vi "Show User Interface.vi"(8 "error in (no error)":errorcluster, 9 "Process VI Refnums":refnum<vi>[](array[refnum]), 10 "Show UI":bool, 11 "SMO.UI":refnum<class "SMO.UI.lvclass">) -> (0 "error out":errorcluster, 3 "SMO.UI out":refnum<class "SMO.UI.lvclass">)   [LabVIEW 2019, in "SMO.UI.lvclass"]
doc: "JKI State Machine Objects (SMO) 1.3.0.56\nJKI - JKI\nCopyright (c) 2017, JKI"
uses:
  SMO.UI.lvclass
  C:/Users/Patrick/Documents/GitHub/Test (LV2019)/lv-venv/lv.lib/vi.lib/JKI/JKI SMO/SMO/SMO.lvclass
  SMO/SMO.lvclass
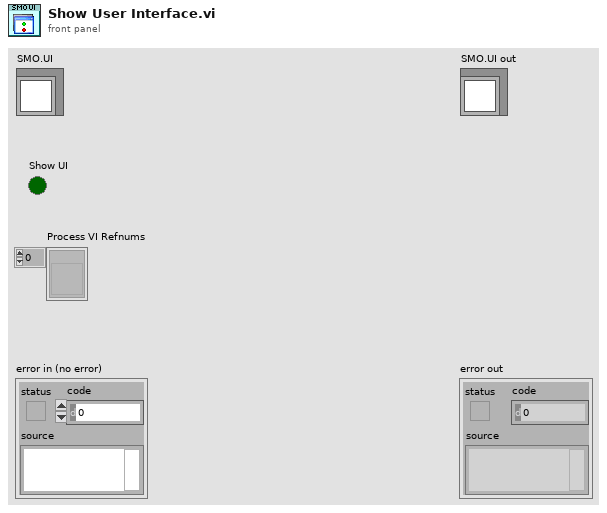
[diagram p1: front panel]
types:
  T1 = enum32{"Invalid", "Standard", "Closed", "Hidden", "Minimized", "Maximized"}
  T2 = typedef "SMO.lvclass/RegisteredProcessData--Cluster.ctl" = cluster{"Name":string, "Static VI Ref":refnum<vi>, "Running":bool, "NotifierRef":u32}
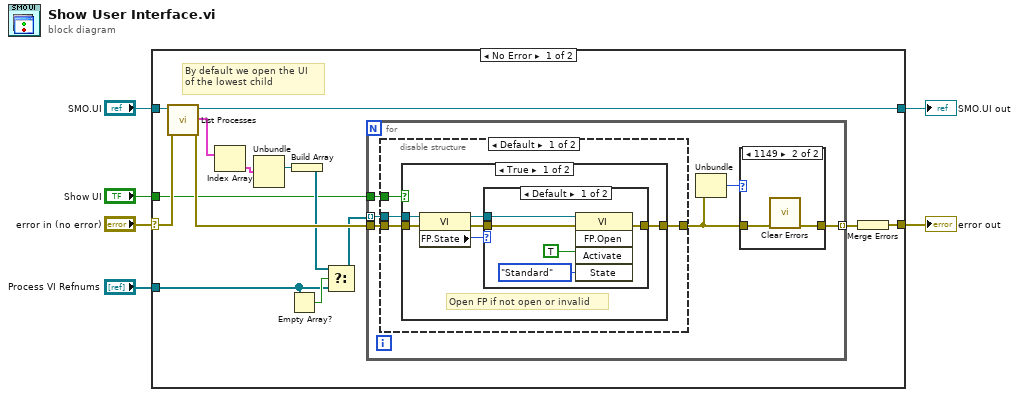
[diagram p0: block diagram]
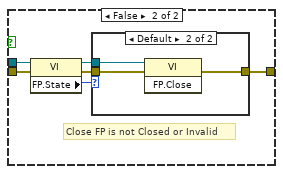
[diagram p4: hidden frame]
diagram:
  n1 = case shown="No Error" "error in (no error)" {
    selector: "error in (no error)" -> [w18 w58]
    tunnel: [w10 w58] -> w5
    tunnel: [w11 w57] -> w3
    tunnel: "SMO.UI" -> [w19 w57]
    tunnel: "Show UI" -> [w9 _]
    tunnel: "Process VI Refnums" -> [w7 _]
    frame No Error {
      # "By default we open the UI \nof the lowest child"
      n2 = call "List Processes.vi"("error in (no error)"=w18, "SMO"=w19) -> ("error out"=w17:errorcluster, "Registered Processes"=w16:T2[], "SMO out"=w11:refnum<class "SMO.UI.lvclass">)  [unwired: 7 in]
      n3 = Index Array(array=w16) -> (element=w15:T2)  [unwired: 1 in]
      n4 = Unbundle(w15) -> ("Static VI Ref"=w12:refnum<vi>)  [unwired: 3 out]
      n5 = Empty Array?(array=w7) -> (empty?=w14:bool)
      n6 = Build Array(w12) -> (w13:refnum<vi>[])
      n7 = Select(t=w13, s=w14, f=w7) -> (s? t:f=w8:refnum<vi>[])
      n8 = for {
        tunnel: w9 -> [w26]
        tunnel: [w21] -> w20 mode=indexing
        tunnel: w8 -> [w25] mode=indexing
        tunnel: w17 -> [w24]
        n9 = disable-structure shown="Default" {
          disable-tunnel: w24 -> [w33 w56]
          disable-tunnel: [w32 w56] -> w22
          disable-tunnel: w25 -> [w31 _]
          disable-tunnel: w26 -> [w30 _]
          frame condition #0 (active) {
            n10 = case shown="True" w30 {
              tunnel: w33 -> [w37 w50]
              tunnel: [w39 w51] -> w32
              tunnel: w31 -> [w38 w48]
              frame True {
                # "Open FP if not open or invalid"
                n11 = property class="VI"(reference=w38, error in=w37) -> (reference out=w35:refnum<vi>, error out=w36:errorcluster, "FP.State"=w34:T1)
                n12 = case shown="Default" w34 {
                  tunnel: [w42 w45] -> w39
                  tunnel: w36 -> [w41 w45]
                  tunnel: w35 -> [w40 _]
                  frame Default {
                    n13 = invoke class="VI" method="FP.Open"(reference=w40, error in=w41, "Activate"=TRUE, "State"=T1."Standard") -> (error out=w42:errorcluster)  [unwired: 1 in, 4 out]
                  }
                  frame "Invalid", "Standard" {
                  }
                }
              }
              frame False {
                # "Close FP is not Closed or Invalid"
                n14 = property class="VI"(reference=w48, error in=w50) -> (reference out=w47:refnum<vi>, error out=w49:errorcluster, "FP.State"=w46:T1)
                n15 = case shown="Default" w46 {
                  tunnel: [w52 w55] -> w51
                  tunnel: w49 -> [w52 w54]
                  tunnel: w47 -> [_ w53]
                  frame "Invalid", "Closed" {
                  }
                  frame Default {
                    n16 = invoke class="VI" method="FP.Close"(reference=w53, error in=w54) -> (error out=w55:errorcluster)  [unwired: 1 in, 2 out]
                  }
                }
              }
            }
          }
          frame condition #1 {
          }
        }
        n17 = Unbundle(w22) -> ("code"=w23:i32)  [unwired: 2 out]
        n18 = case shown="1149" w23 {
          tunnel: [w27 w29] -> w21
          tunnel: w22 -> [w27 w28]
          frame Default {
          }
          frame 1149 {
            n19 = call <vilib>:"Clear Errors.vi"("error in (no error)"=w28) -> ("error out"=w29:errorcluster)  [unwired: 5 in, 1 out]
          }
        }
      }
      n20 = Merge Errors(w20) -> (w10:errorcluster)
    }
    frame Error {
    }
  }
  "error out" <- w5
  "SMO.UI out" <- w3
